vi "PhysionetSignalReader.vi"(8 "error in (no error)":errorcluster, 10 "Convert from ADC units (T)":bool=TRUE, 11 "Header file path":path=path "C:/Users/Andrzej/Desktop/Dropbox/SharedForDADMProj/sygnały/100.hea") -> (0 "error out":errorcluster, 1 "Signals Specs Info":T2[](array[typedef]), 2 "Record Line info":T1, 3 "Signals(physical units)":waveform(dbl)[](array[waveform]), 4 "Signals(ADC units)":i16[][](array[numeric]))   [LabVIEW 2012]
doc: "Reads all information from a Physionet record, which .hea file is given in <b>Header file path</b>. Assumes all of them are in a single binary file, which must be in the same directory as the header file. Supported formats: 212 and 16. If <b>Convert from ADC units</b> is TRUE, samples are converted from raw I16 values to real-world units using data read from header file. Elsewhere, <b>Signals(physical units)</b> is an empty array and raw data is returned in <b>Signals(ADC units)</b>."
uses:
  #TD_SignalSpecInfo.ctl
  #TD_RecordLineInfo.ctl
panel:
  out "Init vals correct":bool[](array[boolean])
  out "Checksums correct":bool[](array[boolean])
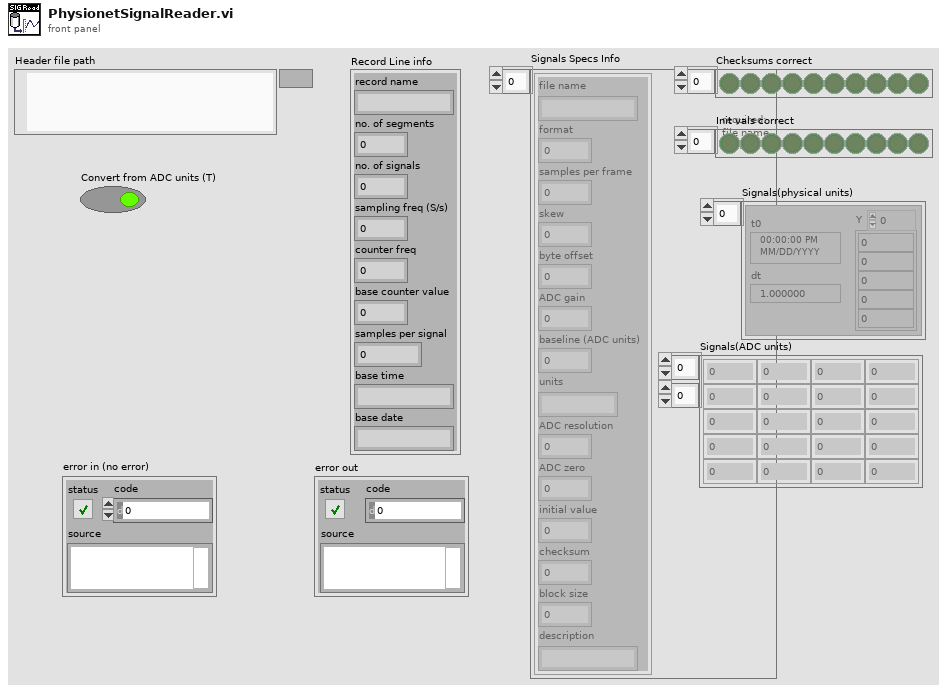
[diagram p1: front panel]
types:
  T1 = typedef "#TD_RecordLineInfo.ctl" = cluster{"record name":string, "no. of segments":i32, "no. of signals":i32, "sampling freq (S/s)":dbl, "counter freq":dbl, "base counter value":dbl, "samples per signal":i32, "base time":string, "base date":string}
  T2 = typedef "#TD_SignalSpecInfo.ctl" = cluster{"file name":string, "format":i32, "samples per frame":i32, "skew":i32, "byte offset":i32, "ADC gain":dbl, "baseline (ADC units)":i16, "units":string, "ADC resolution":i16, "ADC zero":i16, "initial value":i16, "checksum":i16, "block size":i32, "description":string}
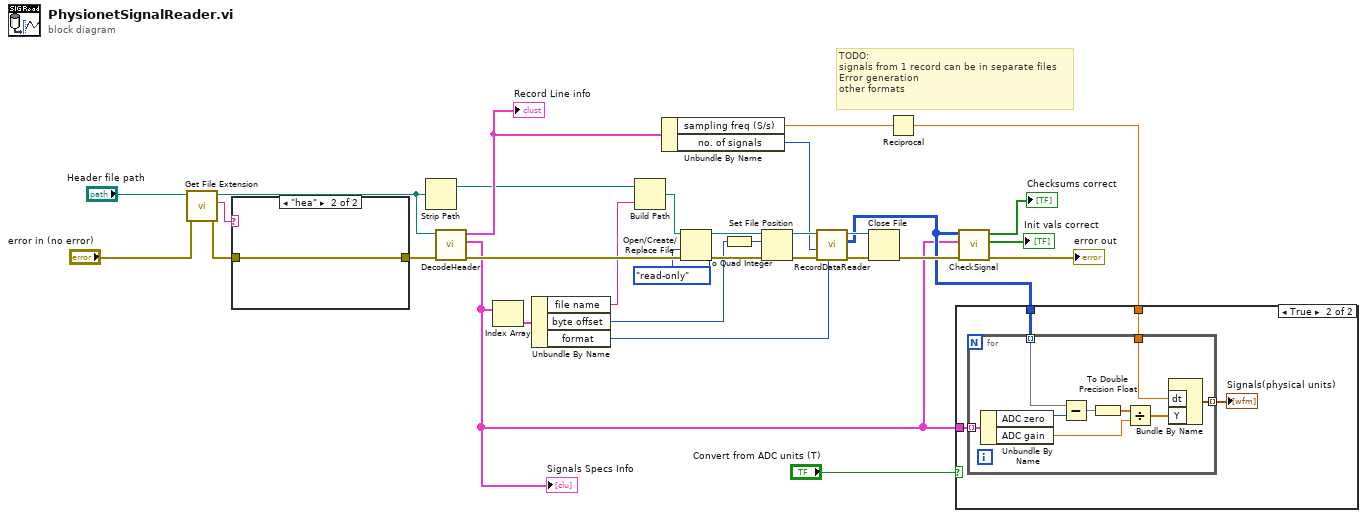
[diagram p0: block diagram]
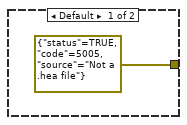
[diagram p2: hidden frame]
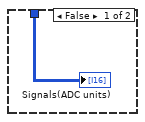
[diagram p3: hidden frame]
diagram:
  # "TODO:\nsignals from 1 record can be in separate files\nError generation\nother formats"
  n1 = call <vilib>:"Get File Extension.vi"("error in (no error)"="error in (no error)", "file"="Header file path") -> ("error out"=w2:errorcluster, "lowercase file extension"=w3:string, "dup file"=w5:path)  [unwired: 6 in, 1 out]
  n2 = case shown="\"hea\"" w3 {
    tunnel: w2 -> [_ w34]
    tunnel: [errorcluster {"status"=TRUE, "code"=5005, "source"="Not a .hea file"} ("error out") w34] -> w1
    frame Default {
    }
    frame "hea" {
    }
  }
  n3 = Strip Path(path=w5) -> (stripped path=w17:path)  [unwired: 1 out]
  n4 = call "DecodeHeader.vi"("error in (no error)"=w1, "Header file path"=w5) -> ("error out"=w31:errorcluster, "Signals Specs Info"=w7:T2[], "Record Line Info"=w32:T1)  [unwired: 4 in, 3 out]
  "Signals Specs Info" <- w7
  "Record Line info" <- w32
  n5 = Index Array(array=w7) -> (element=w21:T2)  [unwired: 1 in]
  n6 = Unbundle By Name(w21) -> ("file name"=w15:string, "byte offset"=w20:i32, "format"=w19:i32)
  n7 = Build Path(base path=w17, name or relative path=w15) -> (appended path=w16:path)
  n8 = Unbundle By Name(w32) -> ("sampling freq (S/s)"=w23:dbl, "no. of signals"=w18:i32)
  n9 = Open/Create/Replace File(file path (use dialog)=w16, error in=w31, access (0:read/write)=enum16{"read/write", "read-only", "write-only"}."read-only") -> (refnum out=w28:refnum<file>, error out=w26:errorcluster)  [unwired: 3 in, 1 out]
  n10 = To Quad Integer(1:w20) -> (0:w24:i64)
  n11 = Set File Position(offset (in bytes) (0)=w24, refnum=w28, error in=w26) -> (refnum out=w27:refnum<file>, error out=w25:errorcluster)  [unwired: 1 in]
  n12 = call "RecordDataReader.vi"("format"=w19, "error in"=w25, "No of signals(1)"=w18, "File refnum in"=w27) -> ("error out"=w13:errorcluster, "Signals"=w8:i16[][], "File refnum out"=w29:refnum<file>)  [unwired: 5 in]
  n13 = Close File(refnum=w29, error in=w13) -> (error out=w9:errorcluster)  [unwired: 1 out]
  n14 = Reciprocal(x=w23) -> (1/x=w22:dbl)
  n15 = case shown="True" "Convert from ADC units (T)" {
    tunnel: w22 -> [_ w39]
    tunnel: w7 -> [_ w38]
    tunnel: w8 -> [w35 w37]
    frame False {
      "Signals(ADC units)" <- w35
    }
    frame True {
      n16 = for {
        tunnel: w37 -> [w40] mode=indexing
        tunnel: [w48] -> w36 mode=indexing
        tunnel: w39 -> [w47]
        tunnel: w38 -> [w46] mode=indexing
        n17 = Unbundle By Name(w46) -> ("ADC zero"=w42:i16, "ADC gain"=w41:dbl)
        n18 = Subtract(x=w40, y=w42) -> (x-y=w45:i16[])
        n19 = To Double Precision Float(number=w45) -> (double precision float=w44:dbl[])
        n20 = Divide(x=w44, y=w41) -> (x/y=w43:dbl[])
        n21 = Bundle By Name("dt"=w47, "Y"=w43) -> (w48:waveform(dbl))  [unwired: 1 in]
      }
      "Signals(physical units)" <- w36
    }
  }
  n22 = call "CheckSignal.vi"("error in (no error)"=w9, "Signals Specs Info"=w7, "Signals"=w8) -> ("error out"=→"error out":errorcluster, "Init vals correct"=→"Init vals correct":bool[], "Checksums correct"=→"Checksums correct":bool[])  [unwired: 6 in]
